vi "Get Items.vi"(8 "error in":errorcluster, 11 "Ctl Refnum":refnum<vi>) -> (0 "error out":errorcluster, 3 "items array":cluster{"Label":string, "Data":variant}[](array[cluster]))   [LabVIEW 2017]
uses:
  <vilib>/Palette API/Palette Menu/Public Type Define/Items.ctl
  <vilib>/Palette API/Palette Menu/Public Type Define/Item.ctl
  <vilib>/Palette API/Palette Menu/Palette Menu.lvlib
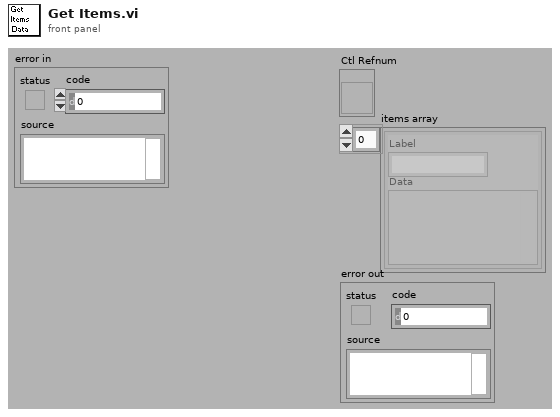
[diagram p1: front panel]
types:
  T1 = typedef "Palette Menu.lvlib/Items.ctl" = T2[]
  T2 = typedef "Palette Menu.lvlib/Item.ctl" = cluster{"item path":path, "library path (.lvlib)":path, "use default lvlib palette":bool, "short name":string, "place VI contents":bool, "hide synchronized item":bool, "reserve spot for synch item":bool, "configure when placing VI contents":bool}
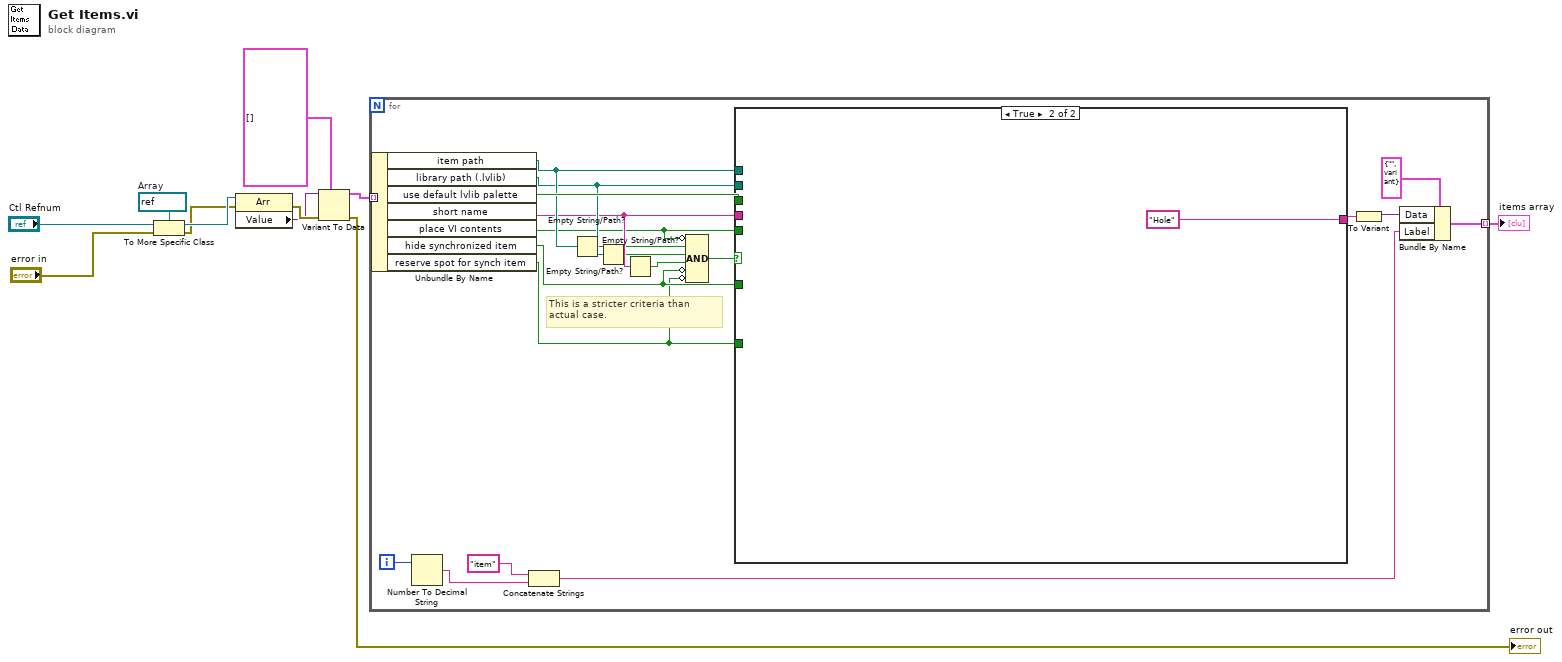
[diagram p0: block diagram]
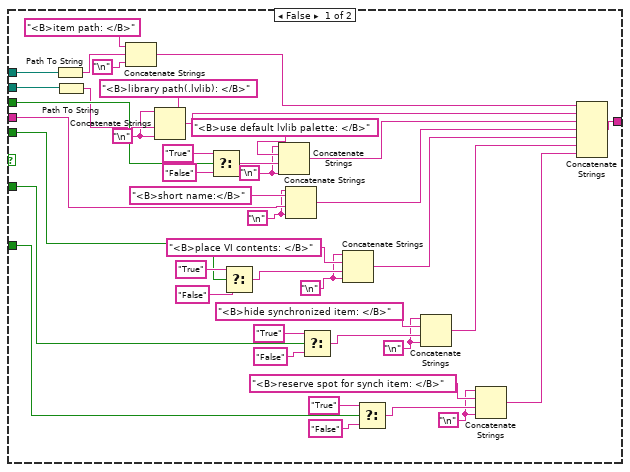
[diagram p2: hidden frame]
diagram:
  w11 = refnum<vi> refnum  # Array
  n1 = To More Specific Class(target class=w11, reference="Ctl Refnum", error in="error in") -> (specific class reference=w10:refnum<vi>, error out=w7:errorcluster)
  n2 = property class="Arr"(reference=w10, error in=w7) -> (error out=w9:errorcluster, "Value"=w8:variant)  [unwired: 1 out]
  n3 = Variant To Data(error in=w9, type=T1 [] ("items"), Variant=w8) -> (data=w5:T1, error out=→"error out":errorcluster)
  n4 = for {
    tunnel: w5 -> [w31] mode=indexing
    tunnel: [w23] -> w3 mode=indexing
    i -> [w26]
    # "This is a stricter criteria than actual case."
    n5 = Unbundle By Name(w31) -> ("item path"=w21:path, "library path (.lvlib)"=w20:path, "use default lvlib palette"=w22:bool, "short name"=w19:string, "place VI contents"=w15:bool, "hide synchronized item"=w14:bool, "reserve spot for synch item"=w13:bool)
    n6 = Number To Decimal String(number=w26) -> (decimal integer string=w25:string)  [unwired: 1 out]
    n7 = Concatenate Strings("item" ("string"), w25) -> (w24:string)
    n8 = Empty String/Path?(string/path=w21) -> (empty?=w18:bool)
    n9 = Empty String/Path?(string/path=w20) -> (empty?=w17:bool)
    n10 = Empty String/Path?(string/path=w19) -> (empty?=w16:bool)
    n11 = Compound Arithmetic op=AND(invert w15, w18, w17, w16, invert w14, invert w13) -> (w12:bool)
    n12 = case shown="True" w12 {
      tunnel: w21 -> [w74 _]
      tunnel: w20 -> [w73 _]
      tunnel: w22 -> [w72 _]
      tunnel: w19 -> [w50 _]
      tunnel: w15 -> [w65 _]
      tunnel: [w59 "Hole"] -> w30
      tunnel: w14 -> [w40 _]
      tunnel: w13 -> [w34 _]
      frame False {
        w35 = "\n"
        w41 = "\n"
        w46 = "\n"
        w48 = "\n"
        w52 = "\n"
        w54 = "\n"
        n13 = Path To String(path=w74) -> (string=w57:string)
        n14 = Path To String(path=w73) -> (string=w69:string)
        n15 = Concatenate Strings("<B>item path: </B>", w57, "\n") -> (w64:string)
        n16 = Concatenate Strings(w54, "<B>library path(.lvlib): </B>" ("element"), w69, w54) -> (w63:string)
        n17 = Select(t="True", s=w72, f="False") -> (s? t:f=w66:string)
        n18 = Select(t="True", s=w65, f="False") -> (s? t:f=w47:string)
        n19 = Concatenate Strings(w52, "<B>use default lvlib palette: </B>" ("element"), w66, w52) -> (w62:string)
        n20 = Concatenate Strings(w48, "<B>short name:</B>" ("element"), w50, w48) -> (w61:string)
        n21 = Select(t="True", s=w40, f="False") -> (s? t:f=w42:string)
        n22 = Concatenate Strings(w46, "<B>place VI contents: </B>" ("element"), w47, w46) -> (w60:string)
        n23 = Select(t="True", s=w34, f="False") -> (s? t:f=w36:string)
        n24 = Concatenate Strings(w41, "<B>hide synchronized item: </B>" ("element"), w42, w41) -> (w33:string)
        n25 = Concatenate Strings(w35, "<B>reserve spot for synch item: </B>" ("element"), w36, w35) -> (w32:string)
        n26 = Concatenate Strings(w64, w63, w62, w61, w60, w33, w32) -> (w59:string)
      }
      frame True {
      }
    }
    n27 = To Variant(anything=w30) -> (Variant=w28:variant)
    n28 = Bundle By Name(cluster=cluster{"Label":string, "Data":variant} {"Label"="", "Data"=variant} ("data cluster"), "Data"=w28, "Label"=w24) -> (w23:cluster{"Label":string, "Data":variant})
  }
  "items array" <- w3
